vi "queue state & data (Single).vi"(6 "Priority Message? (F)":bool, 8 "error in (no error)":errorcluster, 9 "State Data":variant, 10 "State":string, 11 "queue in":refnum<queue>) -> (0 "error out":errorcluster, 3 "queue out":refnum<queue>)   [LabVIEW 2024, in "queue state & data.lvlib"]
uses:
  queue state & data.lvlib
  controls/Message Cluster.ctl
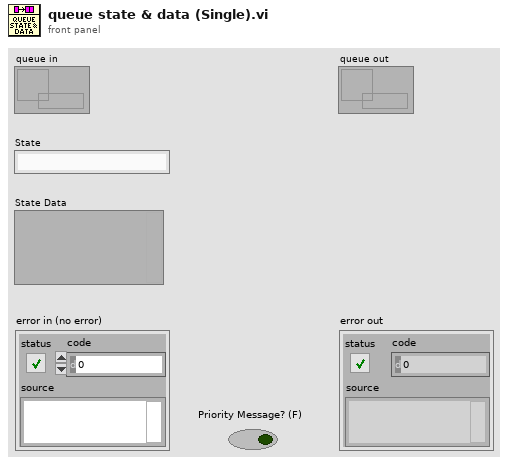
[diagram p1: front panel]
types:
  T1 = typedef "Message Cluster.ctl" = cluster{"Message":string, "Message Data":variant}
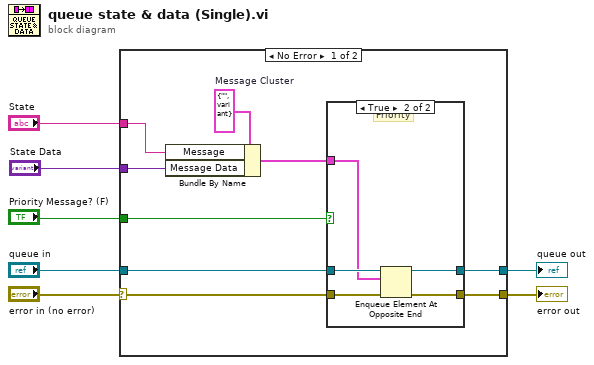
[diagram p0: block diagram]
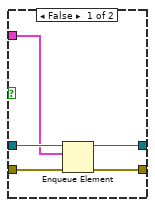
[diagram p2: hidden frame]
diagram:
  n1 = case shown="No Error" "error in (no error)" {
    selector: "error in (no error)" -> [w16 w28]
    tunnel: [w15 w28] -> w6
    tunnel: "State" -> [w13 _]
    tunnel: "Priority Message? (F)" -> [w14 _]
    tunnel: "State Data" -> [w11 _]
    tunnel: [w9 w27] -> w2
    tunnel: "queue in" -> [w8 w27]
    frame No Error {
      w10 = T1 {"Message"="", "Message Data"=variant}  # Message Cluster
      n2 = Bundle By Name(cluster=w10, "Message"=w13, "Message Data"=w11) -> (w12:T1)
      n3 = case shown="True" w14 {
        tunnel: w16 -> [w21 w26]
        tunnel: w12 -> [w17 w22]
        tunnel: [w20 w25] -> w15
        tunnel: [w19 w23] -> w9
        tunnel: w8 -> [w18 w24]
        frame False {
          n4 = Enqueue Element(queue=w18, element=w17, error in (no error)=w21) -> (queue out=w19:refnum<queue>, error out=w20:errorcluster)  [unwired: 1 in, 1 out]
        }
        frame True {
          # "Priority"
          n5 = Enqueue Element At Opposite End(queue=w24, element=w22, error in (no error)=w26) -> (queue out=w23:refnum<queue>, error out=w25:errorcluster)  [unwired: 1 in, 1 out]
        }
      }
    }
    frame Error {
    }
  }
  "error out" <- w6
  "queue out" <- w2
